vi "Reaction_space.vi"(8 "error in":errorcluster, 11 "Input cluster":T1) -> (0 "error out":errorcluster, 1 "Time to react":string, 2 "Reaction space":cluster{dbl[], dbl[]}[](graph), 3 "Ouptut cluster":T1, 5 "OH SHIT BE CAREFUL":bool)   [LabVIEW 2020]
doc: "Update reaction space GUI"
uses:
  controls/StateMachineVariables.ctl
  <vilib>/vision/Avi.llb/IMAQ AVI2 Refnum.ctl
  <vilib>/userDefined/High Color/IMAQdx.ctl
  <vilib>/vision/Deep Learning.llb/IMAQ DL Model Refnum.ctl
  <vilib>/vision/Image Controls.llb/IMAQ Image.ctl
panel:
  out "Speed":dbl format="%#_6p km/h"
  out "clothoid end angle":dbl
  out "clothoid end distance":dbl
  in  "ds":dbl=0.1
  out "Clothoid parameter":dbl
  out "Clothoid length":dbl
  out "Max curve radius":dbl
  out "Braking distance":dbl
  in  "Friction coefficient":dbl=1.0
  out "Car speed m/s":dbl
  in  "Y limit":dbl=6.0
  in  "Car response time":dbl=0.5
  in  "Reaction time":dbl=0.1
  in  "Car width":dbl=2.0
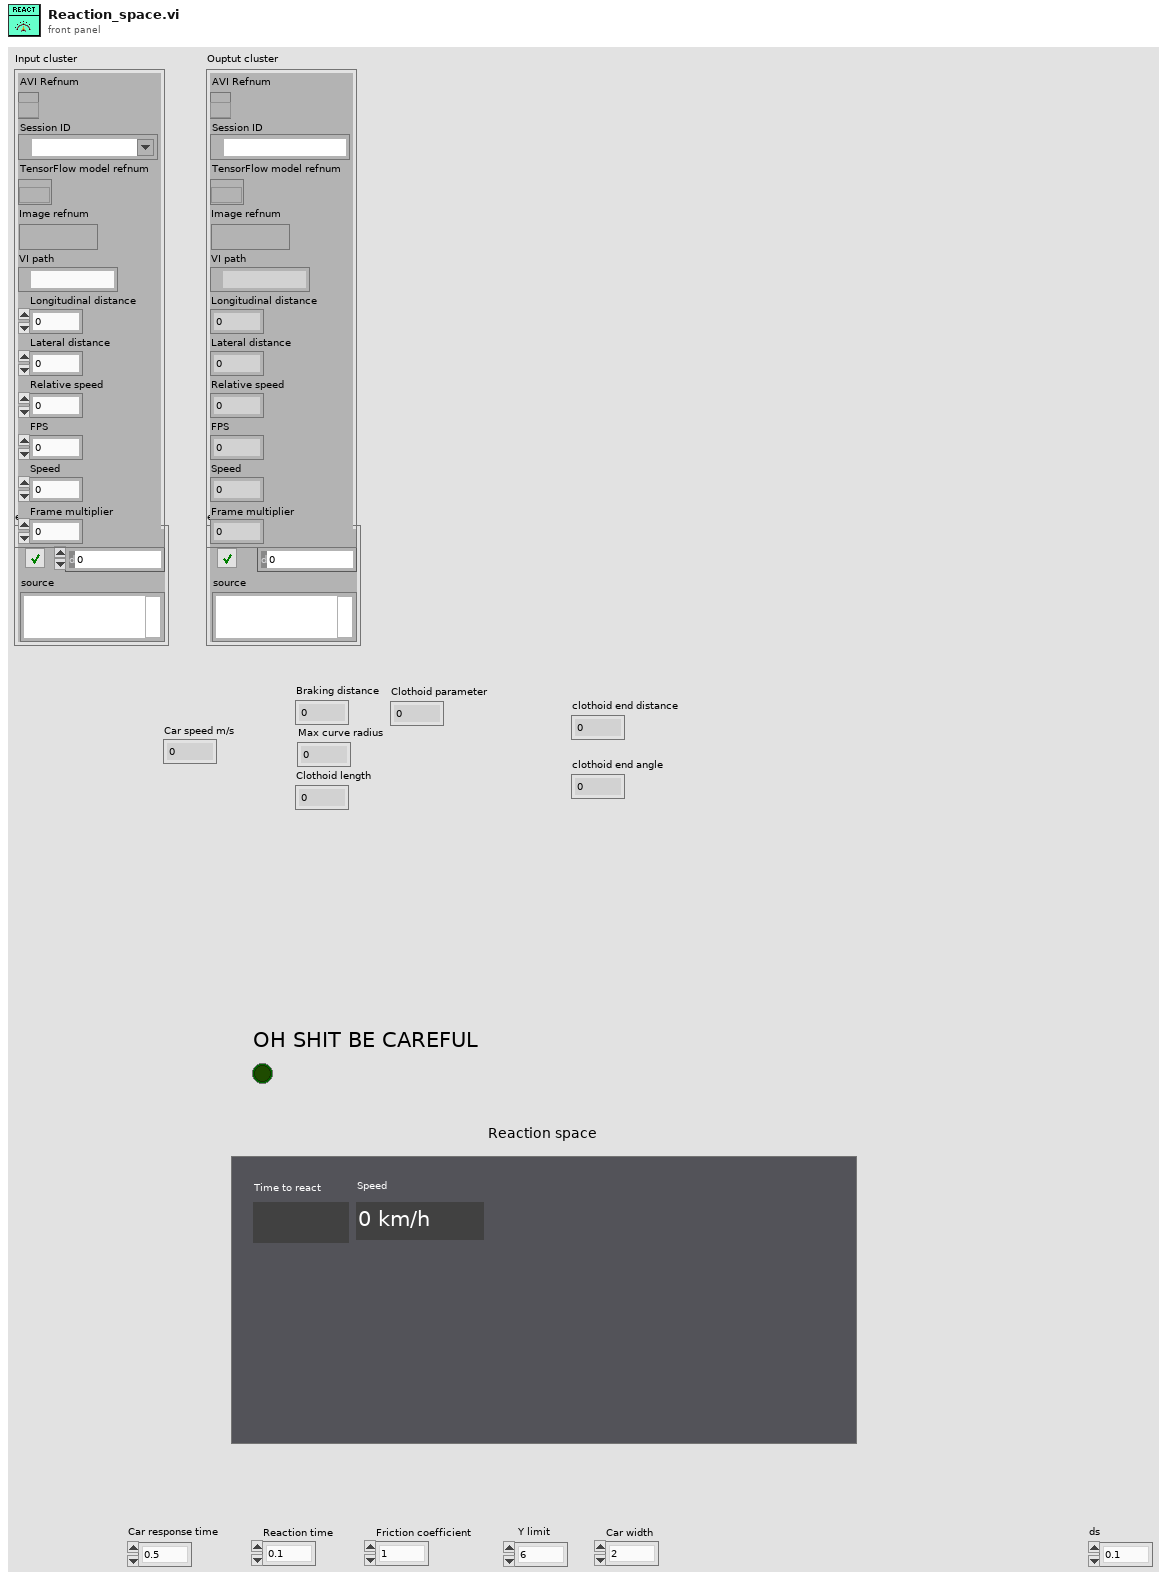
[diagram p1: front panel]
types:
  T1 = typedef "StateMachineVariables.ctl" = cluster{"AVI Refnum":T2, "Session ID":T3, "TensorFlow model refnum":T4, "Image refnum":T5, "VI path":path, "Longitudinal distance":dbl, "Lateral distance":dbl, "Relative speed":dbl, "FPS":dbl, "Speed":dbl, "Frame multiplier":u32}
  T2 = typedef "IMAQ AVI2 Refnum.ctl" = refnum<k20>
  T3 = typedef "IMAQdx.ctl" = refnum<k21>
  T4 = typedef "IMAQ DL Model Refnum.ctl" = refnum<k20>
  T5 = typedef "IMAQ Image.ctl" = refnum<image>
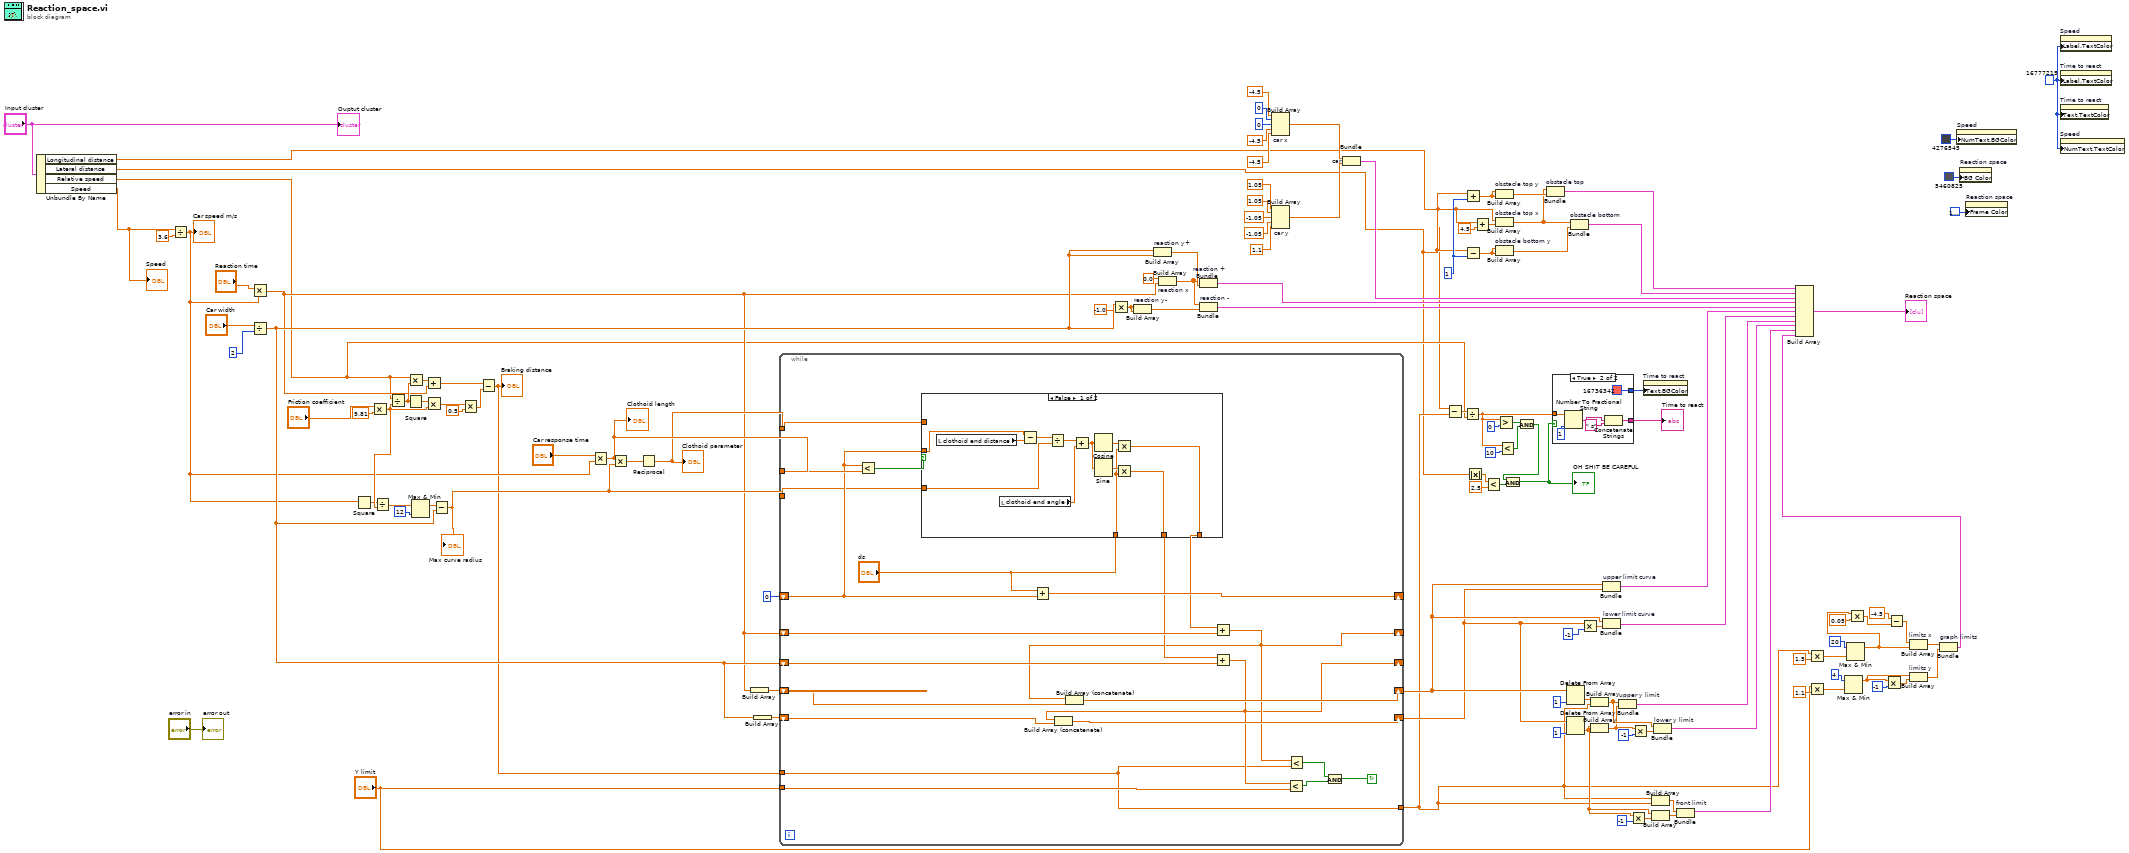
[diagram p0: block diagram]
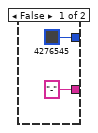
[diagram p2: hidden frame]
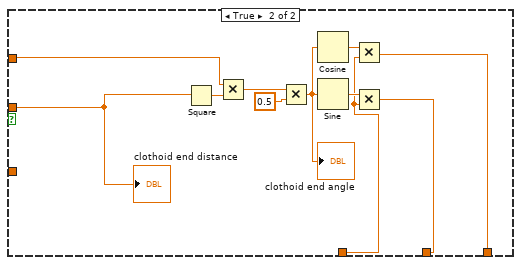
[diagram p3: hidden frame]
diagram:
  w19 = u32 16777215
  w50 = 1
  n1 = Unbundle By Name("Input cluster") -> ("Longitudinal distance"=w5:dbl, "Lateral distance"=w6:dbl, "Relative speed"=w7:dbl, "Speed"=w2:dbl)
  "Speed" <- w2
  n2 = Divide(x=w2, y=3.6) -> (x/y=w41:dbl)
  "Car speed m/s" <- w41
  n3 = Multiply(x="Reaction time", y=w41) -> (x*y=w38:dbl)
  n4 = Divide(x="Car width", y=2) -> (x/y=w92:dbl)
  n5 = Square(x=w41) -> (x^2=w105:dbl)
  n6 = Multiply(x="Friction coefficient", y=9.81) -> (x*y=w106:dbl)
  n7 = Divide(x=w105, y=w106) -> (x/y=w103:dbl)
  n8 = Divide(x=w7, y=w106) -> (x/y=w111:dbl)
  n9 = Square(x=w111) -> (x^2=w110:dbl)
  n10 = Multiply(x=w7, y=w111) -> (x*y=w113:dbl)
  n11 = Max & Min(x=w103, y=12) -> (max(x,y)=w104:dbl)  [unwired: 1 out]
  n12 = Add(x=w113, y=w38) -> (x+y=w112:dbl)
  n13 = Multiply(x=w110, y=w106) -> (x*y=w109:dbl)
  n14 = Subtract(x=w104, y=w92) -> (x-y=w40:dbl)
  "Max curve radius" <- w40
  n15 = Multiply(x=w109, y=0.5) -> (x*y=w107:dbl)
  n16 = Subtract(x=w112, y=w107) -> (x-y=w39:dbl)
  "Braking distance" <- w39
  n17 = Multiply(x="Car response time", y=w41) -> (x*y=w97:dbl)
  "Clothoid length" <- w97
  n18 = Multiply(x=w97, y=w40) -> (x*y=w100:dbl)
  n19 = Reciprocal(x=w100) -> (1/x=w42:dbl)
  "Clothoid parameter" <- w42
  n20 = Build Array(w38) -> (w94:dbl[])
  n21 = Build Array(w92) -> (w93:dbl[])
  n22 = while "s" {
    shift-right: [w130] -> _
    shift-left: w38 -> [w143]
    shift-right: [w129] -> _
    shift-left: w92 -> [w144]
    shift-right: [w142] -> _
    shift-left: 0 -> [w136]
    tunnel: w97 -> [w141]
    tunnel: w40 -> [w135]
    shift-right: [w131] -> w88
    shift-left: w93 -> [w132]
    shift-right: [w133] -> w91
    shift-left: w94 -> [w134]
    tunnel: w42 -> [w128]
    tunnel: "Y limit" -> [w127]
    tunnel: [w126] -> w15
    tunnel: w39 -> [w126]
    stop <- w145 continue-if-true
    n23 = Less?(x=w136, y=w141) -> (x < y?=w140:bool)
    n24 = case shown="False" w140 {
      tunnel: w136 -> [w159 w161]
      tunnel: "ds" -> [w150 w165]
      tunnel: [w149 w164] -> w138
      tunnel: [w148 w163] -> w137
      tunnel: w135 -> [w156 _]
      tunnel: w128 -> [_ w160]
      frame False {
        n25 = local read "clothoid end distance"() -> (w158:dbl)
        n26 = local read "clothoid end angle"() -> (w155:dbl)
        n27 = Subtract(x=w159, y=w158) -> (x-y=w157:dbl)
        n28 = Divide(x=w157, y=w156) -> (x/y=w154:dbl)
        n29 = Add(x=w154, y=w155) -> (x+y=w153:dbl)
        n30 = Cosine(x=w153) -> (cos(x)=w152:dbl)
        n31 = Sine(x=w153) -> (sin(x)=w151:dbl)
        n32 = Multiply(x=w152, y=w150) -> (x*y=w149:dbl)
        n33 = Multiply(x=w151, y=w150) -> (x*y=w148:dbl)
      }
      frame True {
        n34 = Square(x=w161) -> (x^2=w170:dbl)
        n35 = Multiply(x=w160, y=w170) -> (x*y=w169:dbl)
        n36 = Multiply(x=w169, y=0.5) -> (x*y=w162:dbl)
        "clothoid end angle" <- w162
        n37 = Cosine(x=w162) -> (cos(x)=w167:dbl)
        n38 = Sine(x=w162) -> (sin(x)=w166:dbl)
        n39 = Multiply(x=w167, y=w165) -> (x*y=w164:dbl)
        n40 = Multiply(x=w166, y=w165) -> (x*y=w163:dbl)
        "clothoid end distance" <- w161
      }
    }
    n41 = Add(x="ds", y=w136) -> (x+y=w142:dbl)
    n42 = Add(x=w138, y=w143) -> (x+y=w130:dbl)
    n43 = Build Array (concatenate)(w130, w134) -> (w133:dbl[])
    n44 = Add(x=w137, y=w144) -> (x+y=w129:dbl)
    n45 = Build Array (concatenate)(w129, w132) -> (w131:dbl[])
    n46 = Less?(x=w129, y=w127) -> (x < y?=w147:bool)
    n47 = Less?(x=w130, y=w126) -> (x < y?=w146:bool)
    n48 = And(x=w146, y=w147) -> (x .and. y?=w145:bool)
  }
  n49 = Multiply(x=w92, y=-1.0) -> (x*y=w123:dbl)
  n50 = Build Array "reaction y-"(w123, w123) -> (w121:dbl[])
  n51 = Build Array "reaction y+"(w92, w92) -> (w122:dbl[])
  n52 = Build Array "reaction x"(0.0 ("element"), w38) -> (w120:dbl[])
  n53 = Bundle "reaction +"(w120, w122) -> (w119:cluster{dbl[], dbl[]})  [unwired: 1 in]
  n54 = Bundle "reaction -"(w120, w121) -> (w118:cluster{dbl[], dbl[]})  [unwired: 1 in]
  n55 = Build Array "car x"(-4.5, 0, 0, -4.5, -4.5) -> (w66:dbl[])
  n56 = Build Array "car y"(1.05, 1.05, -1.05, -1.05, 1.1) -> (w65:dbl[])
  n57 = Bundle "car"(w66, w65) -> (w64:cluster{dbl[], dbl[]})  [unwired: 1 in]
  n58 = Subtract(x=w5, y=w15) -> (x-y=w25:dbl)
  n59 = Divide(x=w25, y=w7) -> (x/y=w20:dbl)
  n60 = Add(x=w6, y=w50) -> (x+y=w58:dbl)
  n61 = Subtract(x=w6, y=w50) -> (x-y=w54:dbl)
  n62 = Absolute Value(x=w6) -> (abs(x)=w13:dbl)
  n63 = Add(x=w5, y=4.5) -> (x+y=w60:dbl)
  n64 = Less?(x=w13, y=2.5) -> (x < y?=w10:bool)
  n65 = Build Array "obstacle top y"(w58, w58) -> (w59:dbl[])
  n66 = Build Array "obstacle top x"(w5, w60) -> (w55:dbl[])
  n67 = Build Array "obstacle bottom y"(w54, w54) -> (w57:dbl[])
  n68 = Greater?(x=w20, y=0) -> (0:w21:bool)
  n69 = Less?(x=w20, y=10) -> (x < y?=w22:bool)
  n70 = And(x=w21, y=w22) -> (x .and. y?=w11:bool)
  n71 = And(x=w11, y=w10) -> (x .and. y?=w1:bool)
  "OH SHIT BE CAREFUL" <- w1
  n72 = Bundle "obstacle top"(w55, w59) -> (w56:cluster{dbl[], dbl[]})  [unwired: 1 in]
  n73 = case shown="True" w1 {
    tunnel: ["-" w178] -> w18
    tunnel: w20 -> [_ w175]
    tunnel: [u32 4276545 u32 16736342] -> w17
    frame False {
    }
    frame True {
      n74 = Number To Fractional String(number=w175, precision (6)=1) -> (F-format string=w174:string)  [unwired: 2 in]
      n75 = Concatenate Strings(w174, " s") -> (w178:string)
    }
  }
  "Time to react" <- w18
  n76 = Delete From Array(array=w91, index=1) -> (deleted portion=w16:dbl)  [unwired: 1 in, 1 out]
  n77 = Delete From Array(array=w88, index=1) -> (deleted portion=w78:dbl)  [unwired: 1 in, 1 out]
  n78 = Bundle "obstacle bottom"(w55, w57) -> (w53:cluster{dbl[], dbl[]})  [unwired: 1 in]
  n79 = Multiply(x=w88, y=-1) -> (x*y=w96:dbl[])
  n80 = Build Array(w16, w15) -> (w86:dbl[])
  n81 = Build Array(w78, w78) -> (w83:dbl[])
  n82 = Bundle "upper limit curve"(w91, w88) -> (w99:cluster{dbl[], dbl[]})  [unwired: 1 in]
  n83 = Bundle "lower limit curve"(w91, w96) -> (w95:cluster{dbl[], dbl[]})  [unwired: 1 in]
  n84 = Bundle "upper y limit"(w86, w83) -> (w82:cluster{dbl[], dbl[]})  [unwired: 1 in]
  n85 = Multiply(x=w78, y=-1) -> (x*y=w80:dbl)
  n86 = Multiply(x=w83, y=-1) -> (x*y=w84:dbl[])
  n87 = property on="Time to react" class="Str"("Text.BGColor"=w17) -> ()  [unwired: 2 in, 2 out]
  n88 = Build Array(w15, w15) -> (w77:dbl[])
  n89 = Build Array(w78, w80) -> (w76:dbl[])
  n90 = Bundle "lower y limit"(w86, w84) -> (w81:cluster{dbl[], dbl[]})  [unwired: 1 in]
  n91 = Bundle "front limit"(w77, w76) -> (w75:cluster{dbl[], dbl[]})  [unwired: 1 in]
  n92 = Multiply(x=w15, y=1.5) -> (x*y=w43:dbl)
  n93 = Multiply(x="Y limit", y=1.1) -> (x*y=w33:dbl)
  n94 = Max & Min(x=4, y=w33) -> (max(x,y)=w30:dbl)  [unwired: 1 out]
  n95 = Max & Min(x=20, y=w43) -> (max(x,y)=w14:dbl)  [unwired: 1 out]
  n96 = Multiply(x=w14, y=0.05) -> (x*y=w46:dbl)
  n97 = Multiply(x=w30, y=-1) -> (x*y=w29:dbl)
  n98 = Subtract(x=-4.5, y=w46) -> (x-y=w36:dbl)
  n99 = Build Array "limits x"(w36, w14) -> (w27:dbl[])
  n100 = Build Array "limits y"(w30, w29) -> (w28:dbl[])
  n101 = Bundle "graph limits"(w27, w28) -> (w26:cluster{dbl[], dbl[]})  [unwired: 1 in]
  n102 = Build Array(w56, w53, w64, w119, w118, w99, w95, w82, w81, w75, w26) -> (→"Reaction space":cluster{dbl[], dbl[]}[])
  n103 = property on="Speed" class="DigNum (strict)"("NumText.BGColor"=u32 4276545) -> ()  [unwired: 2 in, 2 out]
  n104 = property on="Reaction space" class="XYGraph (strict)"("BG Color"=u32 5460825) -> ()  [unwired: 2 in, 2 out]
  n105 = property on="Reaction space" class="XYGraph (strict)"("Frame Color"=u32 16777216) -> ()  [unwired: 2 in, 2 out]
  n106 = property on="Speed" class="DigNum (strict)"("Label.TextColor"=w19) -> ()  [unwired: 2 in, 2 out]
  n107 = property on="Time to react" class="Str"("Label.TextColor"=w19) -> ()  [unwired: 2 in, 2 out]
  n108 = property on="Time to react" class="Str"("Text.TextColor"=w19) -> ()  [unwired: 2 in, 2 out]
  n109 = property on="Speed" class="DigNum (strict)"("NumText.TextColor"=w19) -> ()  [unwired: 2 in, 2 out]
  "error out" <- "error in"
  "Ouptut cluster" <- "Input cluster"
